vi "HFRR ADV v036 new software.vi"() -> ()   [LabVIEW 2025] (continued)
        n2892 = case shown="True" "OK Button 16" {
          frame False {
          }
          frame True {
            n2893 = stacked-sequence {
              frame #0 {
                n2894 = local read "Numeric 16"() -> (w3957:i32)
                n2895 = local write "Numeric 10"(w3957) -> ()
              }
              frame #1 {
                n2896 = local read "String 29"() -> (w3960:string)
                n2897 = String To Path(string=w3960) -> (path=w3959:path)
                n2898 = Open/Create/Replace File "Open File"(file path (use dialog)=w3959) -> (refnum out=w3961:refnum<file>)  [unwired: 5 in, 2 out]
                n2899 = for {
                  N: 16 -> [_]
                  tunnel: w3961 -> [w3968]
                  i -> [w3964]
                  (unwired) TRUE ("line mode (F)")
                  n2900 = Read from Text File "Read File"(file (use dialog)=w3968) -> (text=w3962:string)  [unwired: 3 in, 3 out]
                  n2901 = Match Pattern(string=w3962, regular expression="(") -> (after substring=w3967:string)  [unwired: 1 in, 3 out]
                  n2902 = Match Pattern(string=w3967, regular expression=")") -> (before substring=w3963:string)  [unwired: 1 in, 3 out]
                  n2903 = case shown="1" w3964 {
                    tunnel: w3963 -> [w3969 w3970 _ _ w3971 w3972 w3973 w3975 w3977 w3979 w3981 w3983 w3985 w3987 _]
                    tunnel: w3962 -> [_ _ _ _ _ _ _ _ _ _ _ _ _ _ _]
                    frame 0 {
                      "TITTLE" <- w3969
                    }
                    frame 1 {
                      "Sample ID" <- w3970
                    }
                    frame 2 {
                    }
                    frame 3 {
                    }
                    frame 4 {
                      "Test Date" <- w3971
                    }
                    frame 5 {
                      "Tested by" <- w3972
                    }
                    frame 6 {
                      n2904 = Fract/Exp String To Number(string=w3973) -> (number=→"Humidity before test 2":dbl)  [unwired: 3 in, 1 out]
                    }
                    frame 7 {
                      n2905 = Fract/Exp String To Number(string=w3975) -> (number=→"Temperature before test 2":dbl)  [unwired: 3 in, 1 out]
                    }
                    frame 8 {
                      n2906 = Fract/Exp String To Number(string=w3977) -> (number=→"Humidity after test 2":dbl)  [unwired: 3 in, 1 out]
                    }
                    frame 9 {
                      n2907 = Fract/Exp String To Number(string=w3979) -> (number=→"Temperature after test 2":dbl)  [unwired: 3 in, 1 out]
                    }
                    frame 10 {
                      n2908 = Fract/Exp String To Number(string=w3981) -> (number=→"MWSD 2":dbl)  [unwired: 3 in, 1 out]
                    }
                    frame 11 {
                      n2909 = Fract/Exp String To Number(string=w3983) -> (number=→"AVP 2":dbl)  [unwired: 3 in, 1 out]
                    }
                    frame 12 {
                      n2910 = Fract/Exp String To Number(string=w3985) -> (number=→"HCF 2":dbl)  [unwired: 3 in, 1 out]
                    }
                    frame 13 {
                      n2911 = Fract/Exp String To Number(string=w3987) -> (number=→"WS1.4 2":dbl)  [unwired: 3 in, 1 out]
                    }
                    frame 14, Default {
                    }
                  }
                }
              }
              frame #2 {
              }
            }
            n2912 = local write "OK Button 16"(FALSE ("OK Button 13")) -> ()
          }
        }
        n2913 = Index Array(array=w3632, index="Select Printer 3") -> (element=w3634:string)
        "Selected Printer" <- w3634
        n2914 = case shown="True" w3629 {
          frame False {
          }
          frame True {
            n2915 = flat-sequence {
              frame #0 {
              }
              frame #1 {
                n2916 = Wait (ms)(milliseconds to wait=u32 100) -> ()  [unwired: 1 out]
              }
              frame #2 {
                n2917 = local write "OK Button 16"(FALSE ("Print 3")) -> ()
              }
            }
          }
        }
        n2918 = case shown="True" "Print" {
          tunnel: w3634 -> [_ w3926]
          frame False {
          }
          frame True {
            (unwired) i16 6 ("width (-)")
            (unwired) "TESTED BY : "
            (unwired) "TESTED DATE :"
            (unwired) "SAMPLE ID : "
            (unwired) "SAMPLE DESIGN : "
            w3884 = "\r"
            w3901 = "\r"
            # "add image"
            n2919 = local read "Sample ID"() -> (w3874:string)
            n2920 = local read "Tested by"() -> (w3877:string)
            n2921 = local read "String 34"() -> (w3864:string)
            n2922 = local read "String 45"() -> (w3844:string)
            n2923 = local read "String 35"() -> (w3859:string)
            n2924 = local read "String 37"() -> (w3857:string)
            n2925 = local read "String 32"() -> (w3879:string)
            n2926 = local read "String 36"() -> (w3854:string)
            n2927 = local read "String 31"() -> (w3878:string)
            n2928 = local read "Test Date"() -> (w3875:string)
            n2929 = local read "String 33"() -> (w3880:string)
            n2930 = local read "String 38"() -> (w3850:string)
            n2931 = local read "String 39"() -> (w3847:string)
            n2932 = local write "Print"(FALSE ("Print FF")) -> ()
            n2933 = local read "S 39"() -> (w3862:string)
            n2934 = local read "S 38"() -> (w3869:string)
            n2935 = local read "Temperature before test 2"() -> (w3900:dbl)
            n2936 = local read "Temperature after test 2"() -> (w3890:dbl)
            n2937 = local read "Humidity before test 2"() -> (w3915:dbl)
            n2938 = local read "Humidity after test 2"() -> (w3899:dbl)
            n2939 = local read "MWSD 2"() -> (w3904:dbl)
            n2940 = local read "WS1.4 2"() -> (w3882:dbl)
            n2941 = Concatenate Strings("2)" ("string"), w3864) -> (w3865:string)
            n2942 = Concatenate Strings("3)" ("string"), w3862) -> (w3863:string)
            n2943 = Concatenate Strings("1)" ("string"), w3869) -> (w3868:string)
            n2944 = Concatenate Strings("4)" ("string"), w3859) -> (w3860:string)
            n2945 = Concatenate Strings("5)" ("string"), w3857) -> (w3856:string)
            n2946 = Concatenate Strings("6)" ("string"), w3854) -> (w3853:string)
            n2947 = Concatenate Strings("7)" ("string"), w3850) -> (w3851:string)
            n2948 = Concatenate Strings("8)" ("string"), w3847) -> (w3848:string)
            n2949 = local read "HCF 2"() -> (w3886:dbl)
            n2950 = local read "AVP 2"() -> (w3903:dbl)
            n2951 = local read "s.NO"() -> (w3845:string)
            n2952 = call <vilib>:"New Report.vi"("report type"=enum16{"Standard Report", "HTML"}."Standard Report") -> ("report out"=w3924:refnum<class "NI_report.lvclass">, "error out"=w3923:errorcluster)  [unwired: 13 in]
            n2953 = local read "TITTLE"() -> (w3876:string)
            n2954 = Concatenate Strings(w3901, w3844, w3845, w3901, w3879, w3874, w3901, w3878, w3875, w3901, w3880, w3877, w3901) -> (w3894:string)
            "test by" <- w3894
            n2955 = Number To Fractional String(number=w3900, width (-)=i16 6, precision (6)=i16 2) -> (F-format string=w3889:string)  [unwired: 1 in]
            n2956 = Number To Fractional String(number=w3899, width (-)=i16 6, precision (6)=i16 2) -> (F-format string=w3902:string)  [unwired: 1 in]
            n2957 = Number To Fractional String(number=w3915, width (-)=i16 6, precision (6)=i16 2) -> (F-format string=w3920:string)  [unwired: 1 in]
            n2958 = Number To Fractional String(number=w3904, width (-)=i16 6, precision (6)=i16 2) -> (F-format string=w3906:string)  [unwired: 1 in]
            n2959 = Number To Fractional String(number=w3890, width (-)=i16 6, precision (6)=i16 2) -> (F-format string=w3891:string)  [unwired: 1 in]
            n2960 = Number To Fractional String(number=w3903, width (-)=i16 6, precision (6)=i16 2) -> (F-format string=w3905:string)  [unwired: 1 in]
            n2961 = Number To Fractional String(number=w3886, width (-)=i16 6, precision (6)=i16 2) -> (F-format string=w3885:string)  [unwired: 1 in]
            n2962 = Number To Fractional String(number=w3882, precision (6)=i16 2) -> (F-format string=w3881:string)  [unwired: 2 in]
            n2963 = call-dynamic "Set Report Header Text.vi"("report in"=w3924, "center header text"=w3876, "error in (no error)"=w3923) -> ("report out"=w3895:refnum<class "NI_report.lvclass">, "error out"=w3896:errorcluster)  [unwired: 11 in]
            n2964 = Concatenate Strings(w3884, w3868, w3920, w3884, w3865, w3889, w3884, w3863, w3902, w3884, w3860, w3891, w3884, w3856, w3906, w3884, w3853, w3905, w3884, w3851, w3885, w3884, w3848, w3881) -> (w3872:string)
            "export 2" <- w3872
            n2965 = call-poly <vilib>:"Append Report Text.vi"("report in"=w3895, "text"=w3894, "error in (no error)"=w3896) -> ("report out"=w3898:refnum<class "NI_report.lvclass">, "error out"=w3897:errorcluster)  [unwired: 9 in, 2 out]
            n2966 = local read "test by"() -> (w3871:string)
            n2967 = local read "TITTLE"() -> (w3873:string)
            n2968 = call-poly <vilib>:"Append Report Text.vi"("report in"=w3898, "error in (no error)"=w3897) -> ("report out"=w3919:refnum<class "NI_report.lvclass">, "error out"=w3917:errorcluster)  [unwired: 10 in, 2 out]
            n2969 = Concatenate Strings(w3873, w3872, w3871) -> (→"output":string)
            n2970 = call-poly <vilib>:"Append Report Text.vi"("report in"=w3919, "text"=w3872, "error in (no error)"=w3917) -> ("report out"=w3918:refnum<class "NI_report.lvclass">, "error out"=w3916:errorcluster)  [unwired: 9 in, 2 out]
            n2971 = call-dynamic "Print Report.vi"("report in"=w3918, "printer name (default)"=w3926, "error in (no error)"=w3916) -> ("report out"=w3928:refnum<class "NI_report.lvclass">, "error out"=w3929:errorcluster)  [unwired: 11 in]
            n2972 = call-dynamic "Dispose Report.vi"("report in"=w3928, "error in (no error)"=w3929) -> ()  [unwired: 13 in, 1 out]
          }
        }
        n2973 = case shown="True" "Print 2" {
          frame False {
          }
          frame True {
            n2974 = flat-sequence {
              frame #0 {
                n2975 = local read "s.NO"() -> (→"s.NO 2":string)
                n2976 = Wait (ms)(milliseconds to wait=u32 20) -> ()  [unwired: 1 out]
                n2977 = local read "Sample ID  3"() -> (→"Sample ID  6":string)
                n2978 = local read "Sample ID  4"() -> (→"Sample ID  7":string)
                n2979 = local read "Sample ID"() -> (→"Sample ID  2":string)
                n2980 = local read "Tested by"() -> (→"Tested by 2":string)
                n2981 = local read "Test Date"() -> (→"Test Date 2":string)
                n2982 = local read "Humidity after test 3"() -> (→"Humidity after test 4":dbl)
                n2983 = local read "Ref A Test Date :"() -> (→"TITTLE 4":string)
                n2984 = local read "Temperature before test 3"() -> (w3751:dbl)
                n2985 = local read "Temperature before test 3"() -> (→"Temperature after test 5":dbl)
                n2986 = local read "Temperature after test 3"() -> (→"Temperature after test 4":dbl)
                n2987 = local read "Humidity before test 3"() -> (→"Humidity before test 4":dbl)
                n2988 = local write "Temperature before test 3"(w3751) -> ()
                n2989 = local read "image data"() -> (w3742:T16)
                n2990 = String To Path(string="C:\\LAB-IQ\\im\\Temp_resized.jpg") -> (path=w3743:path)
                "path 2" <- w3743
                n2991 = call <vilib>:"Write JPEG File.vi"("image data"=w3742, "path to JPEG file"=w3743) -> ()  [unwired: 8 in, 2 out]
                "Ref A Test Date :" <- "Ref A Test Date :"
                "Ref B Test Date :" <- "Ref B Test Date :"
                "Ref B Scar Value :" <- "Ref B Scar Value :"
                "Ref A Scar Value :" <- "Ref A Scar Value :"
              }
              frame #1 {
                (unwired) HTML_Report_Image_Alignment."MIDDLE" ("alignment (default)")
                w3779 = u16 0 items=["portrait", "landscape"] ("orientation (portrait)")
                (unwired) HTML_Report_Image_Alignment."ABSMIDDLE" ("alignment (default)")
                (unwired) "TESTED BY : "
                (unwired) "TESTED DATE :"
                (unwired) "SAMPLE ID : "
                (unwired) "SAMPLE DESIGN : "
                w3812 = "\r"
                # "add image"
                n2992 = Wait (ms)(milliseconds to wait=u32 20) -> ()  [unwired: 1 out]
                n2993 = local read "Sample ID  2"() -> (w3805:string)
                n2994 = local read "Wear Scar X"() -> (w3777:dbl)
                "Length ( microns ) 2" <- w3777
                n2995 = local read "Wear Scar Y"() -> (w3776:dbl)
                "Wear Scar Y ( microns ) :" <- w3776
                n2996 = local read "Test Date 2"() -> (w3806:string)
                n2997 = local read "Tested by 2"() -> (w3807:string)
                n2998 = local read "String 46"() -> (w3803:string)
                n2999 = local read "String 48"() -> (w3809:string)
                n3000 = local read "String 47"() -> (w3808:string)
                n3001 = local read "String 49"() -> (w3810:string)
                n3002 = local read "String 10"() -> (w3763:string)
                n3003 = local read "s.NO 2"() -> (w3804:string)
                n3004 = Add(x=w3777, y=w3776) -> (x+y=w3775:dbl)
                n3005 = call <vilib>:"New Report.vi"("report type"=enum16{"Standard Report", "HTML"}."HTML") -> ("report out"=w3783:refnum<class "NI_report.lvclass">, "error out"=w3781:errorcluster)  [unwired: 13 in]
                n3006 = Concatenate Strings(w3812, w3803, w3804, w3812, w3809, w3805, w3812, w3808, w3806, w3812, w3810, w3807, w3812) -> (→"test by 2":string)
                n3007 = Concatenate Strings("C:\\LAB-IQ\\Data\\" ("string"), w3763, ".jpg" ("string")) -> ()  [unwired: 1 out]
                n3008 = Divide(x=w3775, y=2.0) -> (x/y=→"Mean Wear ( microns) :":dbl)
                n3009 = call-dynamic "Set Report Orientation.vi"("report in"=w3783, "orientation (portrait)"=w3779, "error in (no error)"=w3781) -> ("report out"=w3782:refnum<class "NI_report.lvclass">, "error out"=w3780:errorcluster)  [unwired: 11 in]
                n3010 = for {
                  N: 5 -> [_]
                  tunnel: w3782 -> [w3833]
                  tunnel: [w3832] -> w3761
                  tunnel: w3780 -> [w3831]
                  tunnel: [w3830] -> w3760
                  n3011 = call-dynamic "Set Report Tab Width.vi"("report in"=w3833, "error in (no error)"=w3831) -> ("report out"=w3832:refnum<class "NI_report.lvclass">, "error out"=w3830:errorcluster)  [unwired: 12 in]
                }
                n3012 = local read "TITTLE"() -> (w3778:string)
                n3013 = call-dynamic "Set Report Header Text.vi"("report in"=w3761, "center header text"=w3778, "error in (no error)"=w3760) -> ("report out"=w3799:refnum<class "NI_report.lvclass">, "error out"=w3798:errorcluster)  [unwired: 11 in]
                n3014 = for {
                  N: 1 -> [_]
                  tunnel: [w3837] -> w3785
                  tunnel: [w3836] -> w3784
                  tunnel: w3799 -> [w3835]
                  tunnel: w3798 -> [w3834]
                  n3015 = call-dynamic "New Report Line.vi"("report in"=w3835, "error in (no error)"=w3834) -> ("report out"=w3837:refnum<class "NI_report.lvclass">, "error out"=w3836:errorcluster)  [unwired: 12 in]
                }
                n3016 = for {
                  N: 2 -> [_]
                  tunnel: [w3829] -> w3791
                  tunnel: [w3828] -> w3790
                  tunnel: w3785 -> [w3827]
                  tunnel: w3784 -> [w3826]
                  n3017 = call-dynamic "New Report Line.vi"("report in"=w3827, "error in (no error)"=w3826) -> ("report out"=w3829:refnum<class "NI_report.lvclass">, "error out"=w3828:errorcluster)  [unwired: 12 in]
                }
                n3018 = for {
                  N: 25 -> [_]
                  tunnel: w3791 -> [w3825]
                  tunnel: w3790 -> [w3823]
                  tunnel: [w3824] -> w3794
                  tunnel: [w3822] -> w3793
                  n3019 = call-dynamic "Set Report Tab Width.vi"("report in"=w3825, "error in (no error)"=w3823) -> ("report out"=w3824:refnum<class "NI_report.lvclass">, "error out"=w3822:errorcluster)  [unwired: 12 in]
                }
                n3020 = control-ref of="Tab Control 9"() -> (w3789:refnum<vi>)
                n3021 = call-dynamic "Append Control Image to Report.vi"("report in"=w3794, "alignment (default)"=HTML_Report_Image_Alignment."ABSMIDDLE", "ctrl reference"=w3789, "error in (no error)"=w3793) -> ("report out"=w3788:refnum<class "NI_report.lvclass">, "error out"=w3787:errorcluster)  [unwired: 8 in, 2 out]
                n3022 = for {
                  N: 3 -> [_]
                  tunnel: [w3821] -> w3772
                  tunnel: [w3820] -> w3771
                  tunnel: w3788 -> [w3819]
                  tunnel: w3787 -> [w3818]
                  n3023 = call-dynamic "New Report Line.vi"("report in"=w3819, "error in (no error)"=w3818) -> ("report out"=w3821:refnum<class "NI_report.lvclass">, "error out"=w3820:errorcluster)  [unwired: 12 in]
                }
                n3024 = for {
                  N: 100 -> [_]
                  tunnel: w3772 -> [w3817]
                  tunnel: w3771 -> [w3815]
                  tunnel: [w3816] -> w3768
                  tunnel: [w3814] -> w3766
                  n3025 = call-dynamic "Set Report Tab Width.vi"("report in"=w3817, "error in (no error)"=w3815) -> ("report out"=w3816:refnum<class "NI_report.lvclass">, "error out"=w3814:errorcluster)  [unwired: 12 in]
                }
                n3026 = String To Path(string="C:\\LAB-IQ\\im\\Temp_resized.jpg") -> (path=w3758:path)
                n3027 = call-poly <vilib>:"Append Image to Report.vi"("report in"=w3768, "path or URL of image"=w3758, "error in (no error)"=w3766) -> ("report out"=w3767:refnum<class "NI_report.lvclass">, "error out"=w3765:errorcluster)  [unwired: 9 in, 2 out]
                n3028 = call-poly <vilib>:"Open HTML Report in Browser.vi"("report in"=w3767, "error in (no error)"=w3765) -> ("report out"=w3802:refnum<class "NI_report.lvclass">, "error out"=w3801:errorcluster)  [unwired: 11 in, 1 out]
                n3029 = call-dynamic "Dispose Report.vi"("report in"=w3802, "error in (no error)"=w3801) -> ()  [unwired: 13 in, 1 out]
              }
              frame #2 {
              }
              frame #3 {
                n3030 = disable-structure shown="Disabled" {
                  frame Disabled {
                    n3031 = local read "String 10"() -> (w3842:string)
                    n3032 = Concatenate Strings("C:\\LAB-IQ-NXT\\Data\\" ("string"), w3842, ".jpg" ("string")) -> (w3840:string)
                    n3033 = String To Path(string=w3840) -> (path=w3839:path)
                    n3034 = Delete(path (use dialog)=w3839) -> ()  [unwired: 4 in, 3 out]
                  }
                  frame Enabled {
                  }
                }
                n3035 = local write "Print 2"(FALSE ("Print")) -> ()
              }
            }
          }
        }
      }
    }
    n3036 = Wait (ms)(milliseconds to wait=u32 50) -> ()  [unwired: 1 out]
    n3037 = Wait (ms)(milliseconds to wait=u32 50) -> ()  [unwired: 1 out]
    n3038 = local read "Quit"() -> (w2176:bool)
  }
  n3039 = VISA Close(VISA resource name=w41, error in (no error)=w40) -> ()  [unwired: 1 out]
  n3040 = while {
    stop <- w3993 stop-if-true
    n3041 = local read "Auto Start Test"() -> (w3991:bool)
    n3042 = local read "RUN"() -> (w3990:bool)
    n3043 = Wait (ms)(milliseconds to wait=u32 1000) -> ()  [unwired: 1 out]
    n3044 = Or(x=w3990, y=w3991) -> (x .or. y?=w3989:bool)
    n3045 = case shown="True" w3989 {
      frame False {
      }
      frame True {
        n3046 = local read "LVDT STROKE Actual"() -> (w3994:dbl)
        n3047 = In Range and Coerce(upper limit=1.2, x=w3994, lower limit=0.6) -> (In Range?=w3997:bool)  [unwired: 1 out]
        n3048 = call-poly <vilib>:"Random Number (Range).vi"("lower bound (0)"=0.998 ("upper bound (100)"), "upper bound (100)"=1.003) -> ("number"=w3995:dbl)  [unwired: 9 in]
        n3049 = case shown="True" w3997 {
          tunnel: [w4002 w4003] -> w3996
          tunnel: w3995 -> [_ w4003]
          tunnel: w3994 -> [w4002 _]
          frame False {
          }
          frame True {
          }
        }
        "LVDT STROKE DISPLAY" <- w3996
      }
    }
    n3050 = local read "Quit"() -> (w3993:bool)
  }
  n3051 = while {
    tunnel: [w4020] -> w49
    shift-right: [w4013] -> _
    shift-left: 0.0 -> [w4016]
    shift-right: [w4012] -> _
    shift-left: 0.0 -> [w4015]
    shift-right: [w4011] -> _
    shift-left: 100.0 ("vc_cmd") -> [w4014]
    stop <- w4020 stop-if-true
    # "PID LOGIC"
    n3052 = local read "run test Calibration"() -> (w4008:bool)
    n3053 = local read "RUN"() -> (w4018:bool)
    n3054 = local read "Auto Start Temp"() -> (w4009:bool)
    n3055 = local read "Auto Start Test"() -> (w4017:bool)
    n3056 = local read "START TEMP"() -> (w4007:bool)
    n3057 = And(x=w4009, y=w4017) -> (x .and. y?=w4010:bool)
    n3058 = Or(x=w4018, y=w4010) -> (x .or. y?=w4019:bool)
    n3059 = And(x=w4019, y=w4007) -> (x .and. y?=w4006:bool)
    n3060 = And(x=w4008, y=w4007) -> (x .and. y?=w4005:bool)
    n3061 = Or(x=w4005, y=w4006) -> (x .or. y?=w4004:bool)
    n3062 = Wait (ms)(milliseconds to wait="milliseconds to wait") -> ()  [unwired: 1 out]
    n3063 = case shown="True" w4004 {
      tunnel: [400.0 ("out_vc_cmd") w4039] -> w4011
      tunnel: [w4023 w4041] -> w4012
      tunnel: [w4023 w4040] -> w4013
      tunnel: w4016 -> [_ w4030]
      tunnel: w4015 -> [_ w4029]
      tunnel: w4014 -> [_ w4028]
      tunnel: w4008 -> [_ w4024]
      frame False {
        w4023 = 0.0 ("error_out")
      }
      frame True {
        n3064 = case shown="True" w4024 {
          tunnel: [w4048 1.0] -> w4026
          frame False {
            n3065 = local read "Set Strk"() -> (w4047:dbl)
            n3066 = Add(x=w4047, y="Add up Stroke") -> (x+y=w4048:dbl)
          }
          frame True {
          }
        }
        n3067 = local read "LVDT STROKE"() -> (w4025:dbl)
        n3068 = formula code="// Zero-Hardcode Explicit Positional-Form PID Engine\n// Inputs: target_stroke, measured_stroke, dt, prev_error, integral_accumulator_in, prev_vc_cmd\n//         kp, ki, kd, max_step_change, max_amplitude, min_amplitude, startup_cmd\n// Outputs: vc_cmd, error_out, out_error, integral_accumulator_out, out_vc_cmd\n\n// 1. Calculate Tracking Error\nfloat current_error = target_stroke - measured_stroke;\nerror_out = current_error;\n\n// 2. Compute Proportional Term\nfloat p_term = kp * current_error;\n\n// 3. Compute Derivative Term\nfloat d_term = 0.0;\nif (dt > 0.0) {\n    d_term = kd * ((current_error - prev_error) / dt);\n}\n\n// 4. Update and Accumulate Integral Term\nfloat current_integral = integral_accumulator_in + (current_error * dt);\nfloat i_term = ki * current_integral;\n\n// 5. Calculate Ideal Target Command (Anchored by startup baseline)\nfloat ideal_command = startup_cmd + p_term + i_term + d_term;\n\n// 6. Apply Loop Rate Limiting FIRST \n// (Forces the command to climb gradually from prev_vc_cmd instead of jumping straight to max)\nfloat raw_adjustment = ideal_command - prev_vc_cmd;\n\nif (raw_adjustment > max_step_change) {\n    raw_adjustment = max_step_change;\n} else if (raw_adjustment < -max_step_change) {\n    raw_adjustment = -max_step_change;\n}\n\nfloat next_vc_cmd = prev_vc_cmd + raw_adjustment;\n\n// 7. Anti-Windup Protection & Final Output Safety Safeguard Clamping\n// (Back-calculating based on what we are ACTUALLY outputting)\nif (next_vc_cmd > max_amplitude) {\n    float excess = next_vc_cmd - max_amplitude;\n    if (ki > 0.0) {\n        current_integral -= excess / ki;\n    }\n    next_vc_cmd = max_amplitude;\n} else if (next_vc_cmd < min_amplitude) {\n    float excess = next_vc_cmd - min_amplitude;\n    if (ki > 0.0) {\n        current_integral -= excess / ki;\n    }\n    next_vc_cmd = min_amplitude;\n}\n\n// 8. Map to Shift Registers for memory persistence\nvc_cmd = next_vc_cmd;\nout_error = current_error;                   \nintegral_accumulator_out = current_integral;  \nout_vc_cmd = next_vc_cmd;"("target_stroke"=w4026, "measured_stroke"=w4025, "dt"="dt", "integral_accumulator_in"=w4029, "prev_error"=w4030, "prev_vc_cmd"=w4028, "kp"="kp", "ki"="ki", "kd"="kd", "max_step_change"="max_step_change", "max_amplitude"="max_amplitude", "min_amplitude"="min_amplitude", "startup_cmd"="startup_cmd") -> ("vc_cmd"=w4045:dbl, "out_error"=w4040:dbl, "integral_accumulator_out"=w4041:dbl, "out_vc_cmd"=w4039:dbl)  [unwired: 1 out]
        "output Vpp" <- w4045
        n3069 = Number To Fractional String(number=w4045, precision (6)=i16 1) -> (F-format string=w4043:string)  [unwired: 2 in]
        n3070 = Concatenate Strings("DAC;" ("string"), w4043) -> (w4027:string)
        n3071 = local write "Due Write"(w4027) -> ()
        "prev_error" <- w4030
        "integral_accumulator_in" <- w4029
        "prev_vc_cmd" <- w4028
      }
    }
    n3072 = local read "Quit"() -> (w4020:bool)
  }
  n3073 = Or(x=w45, y=w44) -> (x .or. y?=w46:bool)
  n3074 = Or(x=w42, y=w46) -> (x .or. y?=w51:bool)
  n3075 = control-ref of="new picture"() -> ()  [unwired: 1 out]
  n3076 = Or(x=w54, y=w51) -> (x .or. y?=w48:bool)
  n3077 = Or(x=w48, y=w49) -> (x .or. y?=w43:bool)
  n3078 = while {
    tunnel: [w4050] -> w53
    i -> [w4057]
    stop <- w4050 stop-if-true
    n3079 = local read "Quit"() -> (w4050:bool)
    n3080 = Equal To 0?(x=w4057) -> (x = 0?=w4055:bool)
    n3081 = call "Elapsed Time3"("Time Target (s)"=45.0, "Auto Reset"=TRUE) -> ("Time has Elapsed"=w4054:bool)  [unwired: 10 in, 7 out]
    n3082 = Wait (ms)(milliseconds to wait=u32 50) -> ()  [unwired: 1 out]
    n3083 = Or(x=w4054, y=w4055) -> (x .or. y?=w4056:bool)
    n3084 = case shown="True" w4056 {
      frame False {
      }
      frame True {
        n3085 = call <vilib>:"System Exec.vi"("run minimized? (F)"=TRUE, "error in (no error)"="error in (no error)", "command line"="powercfg.exe -change -monitor-timeout-ac 0") -> ("error out"=w4068:errorcluster)  [unwired: 5 in, 3 out]
        n3086 = call <vilib>:"System Exec.vi"("run minimized? (F)"=TRUE, "error in (no error)"=w4068, "command line"="powercfg.exe -change -disk-timeout-ac 0") -> ("error out"=w4067:errorcluster)  [unwired: 5 in, 3 out]
        n3087 = call <vilib>:"System Exec.vi"("run minimized? (F)"=TRUE, "error in (no error)"=w4067, "command line"="powercfg.exe -change -standby-timeout-ac 0") -> ("error out"=w4066:errorcluster)  [unwired: 5 in, 3 out]
        n3088 = call <vilib>:"System Exec.vi"("run minimized? (F)"=TRUE, "error in (no error)"=w4066, "command line"="powercfg.exe -change -hibernate-timeout-ac 0") -> ("error out"=w4065:errorcluster)  [unwired: 5 in, 3 out]
        n3089 = call <vilib>:"Simple Error Handler.vi"("error in (no error)"=w4065) -> ("error out"=w4071:errorcluster)  [unwired: 4 in, 4 out]
        n3090 = call <vilib>:"Clear Errors.vi"("error in (no error)"=w4071) -> ("error out"=→"error out":errorcluster)  [unwired: 5 in, 1 out]
      }
    }
  }
  n3091 = Compound Arithmetic op=OR(w56, w43, w53) -> (w55:bool)
  n3092 = flat-sequence {
    tunnel: w55 -> [_]
    tunnel: [w4073] -> w25
    tunnel: w25 -> [_]
    frame #0 {
      n3093 = call "CLOSE CONNECTION.vi"() -> ("error out"=w4073:errorcluster)  [unwired: 11 in]
    }
    frame #1 {
      n3094 = Quit LabVIEW(quit? (T)=TRUE) -> ()
      n3095 = local write "Quit"(FALSE ("EXIT")) -> ()
    }
  }
  n3096 = property on="Heater Button" class="Bool (strict)"("Visible"=TRUE) -> ()  [unwired: 2 in, 2 out]
  n3097 = while {
    tunnel: [w4080] -> _
    i -> [w4080]
    stop <- w4076 stop-if-true
    # "Langauage selection"
    n3098 = Equal?(x="Lan flag", y=22.0) -> ()  [unwired: 1 out]
    n3099 = disable-structure shown="Disabled" {
      frame Disabled {
        n3100 = stacked-sequence {
          frame #0 {
            n3101 = case shown="\"Russian\"" "Language Selection" {
              tunnel: [0 1] -> w4082
              frame "English", Default {
              }
              frame "Russian" {
              }
            }
            n3102 = for {
              N: 130 -> [_]
              tunnel: "Table" -> [w4091]
              tunnel: w4082 -> [w4090]
              i -> [w4089]
              n3103 = Index Array(array=w4091, index (row)=w4089, index (col)=w4090) -> (element=w4088:string)
              n3104 = case shown="1" w4089 {
                tunnel: w4088 -> [w4092 w4093 _ w4094 w4095 w4096 w4097 w4098 w4099 w4100 w4101 w4102 w4103 w4104 w4105 w4106 w4107 w4108 w4109 w4110 w4111 w4112 w4113 w4114 w4115 w4116 w4117 w4118 w4119 _ _ w4120 w4121 w4122 w4123 w4124 w4125 w4134 w4141 w4148 w4155 w4159 w4162 w4165 w4167 w4169 w4170 w4171 w4172 w4173 w4174 w4175 w4176 w4177 w4178 w4179 w4180 w4181 w4182 w4183 w4184 w4185 w4186 w4187 w4188 w4189 w4190 w4191 w4192 w4193 w4194 w4195 w4196 w4197 w4198 w4199 w4200 w4201 w4202 w4203 w4204 w4205 w4206 w4207 w4208 w4209 w4210 w4211 w4212 w4213 w4214 w4215 w4216 w4217 w4218 w4219 w4220 w4221 w4222 w4223 w4224 w4225 w4226 w4227 w4228 _ w4229 w4230 w4231 w4232 w4233 w4234 w4235 w4236 w4237 w4238 w4239 w4240 w4241 _ w4242 w4243 w4244 w4245 w4246 w4247 _]
                frame 0 {
                  n3105 = local write "S"(w4092) -> ()
                }
                frame 1 {
                  n3106 = local write "S 2"(w4093) -> ()
                }
                frame 2 {
                }
                frame 3 {
                  n3107 = local write "S 4"(w4094) -> ()
                }
                frame 4 {
                  n3108 = property on="FILE" class="Str"("Caption.Text"=w4095) -> ()  [unwired: 2 in, 2 out]
                }
                frame 5 {
                  n3109 = property on="Fuel Discription :" class="Str"("Caption.Text"=w4096) -> ()  [unwired: 2 in, 2 out]
                }
                frame 6 {
                  n3110 = property on="Remarks :" class="Str"("Caption.Text"=w4097) -> ()  [unwired: 2 in, 2 out]
                }
                frame 7 {
                  n3111 = property on="Save & Continue" class="Bool (strict)"("Boolean Text.Text"=w4098) -> ()  [unwired: 2 in, 2 out]
                }
                frame 8 {
                }
                frame 9 {
                  n3112 = property on="Set Hz" class="DigNum (strict)"("Caption.Text"=w4100) -> ()  [unwired: 2 in, 2 out]
                }
                frame 10 {
                }
                frame 11 {
                  n3113 = property on="NORMAL LOAD" class="DigNum (strict)"("Caption.Text"=w4102) -> ()  [unwired: 2 in, 2 out]
                }
                frame 12 {
                }
                frame 13 {
                  n3114 = property on="Set Temp" class="DigNum (strict)"("Caption.Text"=w4104) -> ()  [unwired: 2 in, 2 out]
                }
                frame 14 {
                  n3115 = local write "S 15"(w4105) -> ()
                }
                frame 15 {
                  n3116 = property on="Set Rh" class="DigNum (strict)"("Caption.Text"=w4106) -> ()  [unwired: 2 in, 2 out]
                }
                frame 16 {
                }
                frame 17 {
                  n3117 = local write "S 18"(w4108) -> ()
                }
                frame 18 {
                  "String 17" <- w4109
                }
                frame 19 {
                  n3118 = property on="test time" class="DigNum (strict)"("Caption.Text"=w4110) -> ()  [unwired: 2 in, 2 out]
                }
                frame 20 {
                  "String 18" <- w4111
                  "String 22" <- w4111
                }
                frame 21 {
                  n3119 = property on="Elapsed time" class="DigNum (strict)"("Caption.Text"=w4112) -> ()  [unwired: 2 in, 2 out]
                }
                frame 22 {
                  n3120 = property on="Samplingtime 2" class="DigNum (strict)"("Caption.Text"=w4113) -> ()  [unwired: 2 in, 2 out]
                }
                frame 23 {
                  "String 21" <- w4114
                }
                frame 24 {
                  n3121 = property on="Countdown" class="DigNum (strict)"("Caption.Text"=w4115) -> ()  [unwired: 2 in, 2 out]
                }
                frame 25 {
                  n3122 = property on="Countdown 2" class="DigNum (strict)"("Caption.Text"=w4116) -> ()  [unwired: 2 in, 2 out]
                }
                frame 26 {
                  n3123 = property on="Engage" class="Bool (strict)"("Boolean Text.Text"=w4117) -> ()  [unwired: 2 in, 2 out]
                }
                frame 27 {
                  n3124 = property on="Boolean  4" class="Bool (strict)"("Boolean Text.Text"=w4118) -> ()  [unwired: 2 in, 2 out]
                }
                frame 28 {
                  n3125 = property on="Test \nStatus" class="Bool (strict)"("Boolean Text.Text"=w4119) -> ()  [unwired: 2 in, 2 out]
                }
                frame 29 {
                }
                frame 30 {
                }
                frame 31 {
                }
                frame 32 {
                  n3126 = property on="RSTCOF" class="Bool"("Boolean Text.Text"=w4121) -> ()  [unwired: 2 in, 2 out]
                  n3127 = property on="RST FF" class="Bool"("Boolean Text.Text"=w4121) -> ()  [unwired: 2 in, 2 out]
                  n3128 = property on="RST TEMP" class="Bool"("Boolean Text.Text"=w4121) -> ()  [unwired: 2 in, 2 out]
                  n3129 = property on="RSTV1 3" class="Bool"("Boolean Text.Text"=w4121) -> ()  [unwired: 2 in, 2 out]
                  n3130 = property on="rstv2" class="Bool"("Boolean Text.Text"=w4121) -> ()  [unwired: 2 in, 2 out]
                  n3131 = property on="RSTV1 2" class="Bool"("Boolean Text.Text"=w4121) -> ()  [unwired: 2 in, 2 out]
                  n3132 = property on="RST CP" class="Bool"("Boolean Text.Text"=w4121) -> ()  [unwired: 2 in, 2 out]
                }
                frame 33 {
                  "S 61" <- w4122
                }
                frame 34 {
                  "String 23" <- w4123
                }
                frame 35 {
                  n3133 = property on="Rh Before" class="DigNum (strict)"("Caption.Text"=w4124) -> ()  [unwired: 2 in, 2 out]
                }
                frame 36 {
                  n3134 = Match Pattern(string=w4125, regular expression=",") -> (before substring=→"bs":string, after substring=→"as":string)  [unwired: 1 in, 2 out]
                  n3135 = property on="Rh After" class="DigNum (strict)"("Caption.Text"=w4125) -> ()  [unwired: 2 in, 2 out]
                }
                frame 37 {
                  n3136 = Match Pattern(string=w4134, regular expression=",") -> (before substring=w4133:string, after substring=w4132:string)  [unwired: 1 in, 2 out]
                  "bs" <- w4133
                  "as" <- w4132
                  n3137 = Concatenate Strings(w4133, w4132) -> (w4129:string)
                  n3138 = property on="Humidity before test 2" class="DigNum (strict)"("Caption.Text"=w4129) -> ()  [unwired: 2 in, 2 out]
                  n3139 = Concatenate Strings(w4129, "=" ("string")) -> (w4130:string)
                  n3140 = local write "S 38"(w4130) -> ()
                }
                frame 38 {
                  n3141 = Match Pattern(string=w4141, regular expression=",") -> (before substring=w4140:string, after substring=w4139:string)  [unwired: 1 in, 2 out]
                  "bs" <- w4140
                  "as" <- w4139
                  n3142 = Concatenate Strings(w4140, w4139) -> (w4136:string)
                  n3143 = property on="Humidity after test 2" class="DigNum (strict)"("Caption.Text"=w4136) -> ()  [unwired: 2 in, 2 out]
                  n3144 = Concatenate Strings(w4136, "=" ("string")) -> (w4138:string)
                  n3145 = local write "S 39"(w4138) -> ()
                }
                frame 39 {
                  n3146 = Match Pattern(string=w4148, regular expression=",") -> (before substring=w4147:string, after substring=w4146:string)  [unwired: 1 in, 2 out]
                  "bs" <- w4147
                  "as" <- w4146
                  n3147 = Concatenate Strings(w4147, w4146) -> (w4143:string)
                  n3148 = property on="Temperature before test 2" class="DigNum (strict)"("Caption.Text"=w4143) -> ()  [unwired: 2 in, 2 out]
                  n3149 = Concatenate Strings(w4143, "=" ("string")) -> (→"String 34":string)
                }
                frame 40 {
                  n3150 = Match Pattern(string=w4155, regular expression=",") -> (before substring=w4154:string, after substring=w4153:string)  [unwired: 1 in, 2 out]
                  "bs" <- w4154
                  "as" <- w4153
                  n3151 = Concatenate Strings(w4154, w4153) -> (w4150:string)
                  n3152 = property on="Temperature after test 2" class="DigNum (strict)"("Caption.Text"=w4150) -> ()  [unwired: 2 in, 2 out]
                  n3153 = Concatenate Strings(w4150, "=" ("string")) -> (→"String 35":string)
                  n3154 = property on="Temperature after test" class="DigNum (strict)"("Caption.Text"=w4150) -> ()  [unwired: 2 in, 2 out]
                }
                frame 41 {
                  n3155 = property on="AVP 2" class="DigNum (strict)"("Caption.Text"=w4159) -> ()  [unwired: 2 in, 2 out]
                  n3156 = Concatenate Strings(w4159, "=" ("string")) -> (→"String 36":string)
                }
                frame 42 {
                  n3157 = property on="MWSD 2" class="DigNum (strict)"("Caption.Text"=w4162) -> ()  [unwired: 2 in, 2 out]
                  n3158 = Concatenate Strings(w4162, "=" ("string")) -> (→"String 37":string)
                }
                frame 43 {
                  n3159 = property on="HCF 2" class="DigNum (strict)"("Caption.Text"=w4165) -> ()  [unwired: 2 in, 2 out]
                  n3160 = Concatenate Strings(w4165, "=" ("string")) -> (→"String 38":string)
                }
                frame 44 {
                  n3161 = Concatenate Strings(w4167, "=" ("string")) -> (→"String 39":string)
                  n3162 = property on="WS1.4 2" class="DigNum (strict)"("Caption.Text"=w4167) -> ()  [unwired: 2 in, 2 out]
                }
                frame 45 {
                }
                frame 46 {
                  n3163 = local write "S 47"(w4170) -> ()
                }
                frame 47 {
                  n3164 = local write "S 48"(w4171) -> ()
                }
                frame 48 {
                  n3165 = local write "S 49"(w4172) -> ()
                }
                frame 49 {
                  n3166 = local write "S 50"(w4173) -> ()
                }
                frame 50 {
                  n3167 = local write "S 51"(w4174) -> ()
                }
                frame 51 {
                  n3168 = local write "S 52"(w4175) -> ()
                }
                frame 52 {
                  n3169 = local write "S 53"(w4176) -> ()
                }
                frame 53 {
                  n3170 = local write "S 54"(w4177) -> ()
                }
                frame 54 {
                  n3171 = local write "S 55"(w4178) -> ()
                }
                frame 55 {
                  n3172 = local write "S 56"(w4179) -> ()
                }
                frame 56 {
                  n3173 = local write "S 57"(w4180) -> ()
                }
                frame 57 {
                  n3174 = local write "S 58"(w4181) -> ()
                }
                frame 58 {
                  n3175 = local write "S 59"(w4182) -> ()
                }
                frame 59 {
                  n3176 = local write "S 60"(w4183) -> ()
                }
                frame 60 {
                  n3177 = local write "S 62"(w4184) -> ()
                }
                frame 61 {
                  n3178 = local write "S 63"(w4185) -> ()
                }
                frame 62 {
                  n3179 = local write "S 64"(w4186) -> ()
                }
                frame 63 {
                  n3180 = local write "S 65"(w4187) -> ()
                }
                frame 64 {
                  n3181 = local write "S 66"(w4188) -> ()
                }
                frame 65 {
                  n3182 = local write "S 67"(w4189) -> ()
                }
                frame 66 {
                  n3183 = local write "S 68"(w4190) -> ()
                }
                frame 67 {
                  n3184 = local write "S 69"(w4191) -> ()
                }
                frame 68 {
                  n3185 = local write "S 70"(w4192) -> ()
                }
                frame 69 {
                  n3186 = local write "S 71"(w4193) -> ()
                }
                frame 70 {
                  n3187 = local write "S 72"(w4194) -> ()
                }
                frame 71 {
                  n3188 = local write "S 73"(w4195) -> ()
                }
                frame 72 {
                  n3189 = local write "S 74"(w4196) -> ()
                }
                frame 73 {
                  n3190 = local write "S 75"(w4197) -> ()
                }
                frame 74 {
                  n3191 = local write "S 76"(w4198) -> ()
                }
                frame 75 {
                  n3192 = local write "S 77"(w4199) -> ()
                }
                frame 76 {
                  n3193 = local write "S 78"(w4200) -> ()
                }
                frame 77 {
                  n3194 = local write "S 79"(w4201) -> ()
                }
                frame 79 {
                  n3195 = property on="Sample Temperature ( °C )" class="XYGraph (strict)"("Y Scale.Name Label.Text"=w4202) -> ()  [unwired: 2 in, 2 out]
                }
                frame 80 {
                  n3196 = local write "S 81"(w4203) -> ()
                  n3197 = property on="Humidity ( %RH )" class="XYGraph (strict)"("Y Scale.Name Label.Text"=w4203) -> ()  [unwired: 2 in, 2 out]
                }
                frame 78 {
                  n3198 = property on="Air Temperature  ( °C )" class="XYGraph (strict)"("X Scale.Name Label.Text"=w4204) -> ()  [unwired: 2 in, 2 out]
                  n3199 = property on="Humidity ( %RH )" class="XYGraph (strict)"("X Scale.Name Label.Text"=w4204) -> ()  [unwired: 2 in, 2 out]
                  n3200 = property on="Sample Temperature ( °C )" class="XYGraph (strict)"("X Scale.Name Label.Text"=w4204) -> ()  [unwired: 2 in, 2 out]
                  n3201 = property on="Coefficient Of Friction" class="XYGraph (strict)"("X Scale.Name Label.Text"=w4204) -> ()  [unwired: 2 in, 2 out]
                }
                frame 81 {
                  n3202 = property on="Air Temperature  ( °C )" class="XYGraph (strict)"("Y Scale.Name Label.Text"=w4205) -> ()  [unwired: 2 in, 2 out]
                }
                frame 82 {
                  n3203 = local write "S 84"(w4206) -> ()
                }
                frame 83 {
                  n3204 = local write "S 85"(w4207) -> ()
                }
                frame 84 {
                  n3205 = local write "S 86"(w4208) -> ()
                }
                frame 85 {
                  n3206 = local write "S 87"(w4209) -> ()
                }
                frame 86 {
                  n3207 = local write "S 88"(w4210) -> ()
                }
                frame 87 {
                }
                frame 88 {
                  n3208 = local write "S 90"(w4212) -> ()
                }
                frame 89 {
                  n3209 = local write "S 91"(w4213) -> ()
                }
                frame 90 {
                  n3210 = local write "S 92"(w4214) -> ()
                }
                frame 91 {
                  n3211 = local write "S 93"(w4215) -> ()
                }
                frame 92 {
                  n3212 = local write "S 94"(w4216) -> ()
                }
                frame 93 {
                  n3213 = local write "S 95"(w4217) -> ()
                }
                frame 94 {
                  n3214 = local write "S 96"(w4218) -> ()
                }
                frame 95 {
                  n3215 = local write "S 97"(w4219) -> ()
                }
                frame 96 {
                  n3216 = local write "S 98"(w4220) -> ()
                }
                frame 97 {
                  n3217 = local write "S 99"(w4221) -> ()
                }
                frame 98 {
                  n3218 = local write "S 100"(w4222) -> ()
                }
                frame 99 {
                  n3219 = local write "S 101"(w4223) -> ()
                }
                frame 100 {
                  n3220 = local write "S 102"(w4224) -> ()
                }
                frame 101 {
                  n3221 = local write "S 103"(w4225) -> ()
                }
                frame 102 {
                  n3222 = local write "S 104"(w4226) -> ()
                }
                frame 103 {
                  n3223 = local write "S 105"(w4227) -> ()
                }
                frame 104 {
                  n3224 = local write "S 106"(w4228) -> ()
                }
                frame 105 {
                }
                frame 106 {
                  n3225 = property on="OK Button 17" class="Bool (strict)"("Boolean Text.Text"=w4229) -> ()  [unwired: 2 in, 2 out]
                }
                frame 107 {
                  n3226 = property on="OK Button 16" class="Bool (strict)"("Boolean Text.Text"=w4230) -> ()  [unwired: 2 in, 2 out]
                }
                frame 108 {
                  n3227 = property on="TITTLE" class="Str"("Caption.Text"=w4231) -> ()  [unwired: 2 in, 2 out]
                }
                frame 109 {
                  "String 30" <- w4232
                }
                frame 110 {
                  n3228 = property on="Test Date" class="Str"("Caption.Text"=w4233) -> ()  [unwired: 2 in, 2 out]
                  "String 31" <- w4233
                }
                frame 111 {
                  n3229 = property on="Sample ID" class="Str"("Caption.Text"=w4234) -> ()  [unwired: 2 in, 2 out]
                  "String 32" <- w4234
                }
                frame 112 {
                  n3230 = property on="Tested by" class="Str"("Caption.Text"=w4235) -> ()  [unwired: 2 in, 2 out]
                  "String 33" <- w4235
                }
                frame 113 {
                  n3231 = property on="System Configured Printers 2" class="Arr (strict)"("Caption.Text"=w4236) -> ()  [unwired: 2 in, 2 out]
                }
                frame 114 {
                  n3232 = property on="Selected Printer" class="Str"("Caption.Text"=w4237) -> ()  [unwired: 2 in, 2 out]
                }
                frame 115 {
                  n3233 = property on="Select Printer 3" class="DigNum (strict)"("Caption.Text"=w4238) -> ()  [unwired: 2 in, 2 out]
                }
                frame 116 {
                  n3234 = property on="Print" class="Bool (strict)"("Boolean Text.Text"=w4239) -> ()  [unwired: 2 in, 2 out]
                }
                frame 117 {
                  "String 41" <- w4240
                }
                frame 118 {
                  n3235 = property on="tested by" class="Str"("Caption.Text"=w4241) -> ()  [unwired: 2 in, 2 out]
                }
                frame 119 {
                }
                frame 120 {
                  n3236 = property on="Export" class="Bool (strict)"("Boolean Text.Text"=w4242) -> ()  [unwired: 2 in, 2 out]
                }
                frame 121 {
                }
                frame 122 {
                }
                frame 123 {
                  n3237 = property on="Select File Type" class="Enum (strict)"("Caption.Text"=w4245) -> ()  [unwired: 2 in, 2 out]
                }
                frame 124 {
                  n3238 = property on="s.NO" class="Str"("Caption.Text"=w4246) -> ()  [unwired: 2 in, 2 out]
                  "String 45" <- w4246
                }
                frame 125 {
                  n3239 = property on="trip1 8" class="Bool (strict)"("Boolean Text.Text"=w4247) -> ()  [unwired: 2 in, 2 out]
                }
                frame 126, Default {
                }
              }
            }
          }
          frame #1 {
            w4255 = TRUE ("Visible")
            n3240 = local read "S 91"() -> (w4272:string)
            n3241 = local read "S 90"() -> (w4271:string)
            n3242 = local read "S 88"() -> (w4270:string)
            n3243 = property on="File Path" class="Path"("Caption.Text"=w4271) -> ()  [unwired: 2 in, 2 out]
            n3244 = local read "S 71"() -> (w4265:string)
            n3245 = local read "S 86"() -> (w4267:string)
            n3246 = local read "S 85"() -> (w4268:string)
            n3247 = local read "S 87"() -> (w4266:string)
            n3248 = local read "S 84"() -> (w4269:string)
            n3249 = local read "S 103"() -> (w4254:string)
            n3250 = local read "S 104"() -> (w4253:string)
            n3251 = property on="Password" class="Str"("Caption.Text"=w4268) -> ()  [unwired: 2 in, 2 out]
            n3252 = property on="EDIT" class="Bool (strict)"("Boolean Text.Text"=w4265) -> ()  [unwired: 2 in, 2 out]
            n3253 = property on="SAVE" class="Bool (strict)"("Boolean Text.Text"=w4269) -> ()  [unwired: 2 in, 2 out]
            n3254 = Build Array(w4254, w4253) -> (w4252:string[])
            n3255 = property on="Heater Button" class="Bool (strict)"("Strings [4]"=w4252) -> ()  [unwired: 2 in, 2 out]
            n3256 = local read "S 92"() -> (w4264:string)
            n3257 = local read "S 93"() -> (w4263:string)
            n3258 = local read "S 105"() -> (w4250:string)
            n3259 = local read "S 106"() -> (w4249:string)
            n3260 = Build Array(w4264, w4263) -> ()  [unwired: 1 out]
            n3261 = Build Array(w4250, w4249) -> (w4251:string[])
            n3262 = local read "S 95"() -> (w4261:string)
            n3263 = local read "S 94"() -> (w4262:string)
            n3264 = local read "bs"() -> (w4277:string)
            n3265 = local read "as"() -> (w4278:string)
            n3266 = property on="Humidity" class="Bool (strict)"("Strings [4]"=w4251) -> ()  [unwired: 2 in, 2 out]
            n3267 = Concatenate Strings(w4277, "\r", w4278) -> ()  [unwired: 1 out]
            n3268 = property on="Rh After" class="DigNum (strict)"("Caption.Size to Text?"=TRUE ("Caption.Size to Text")) -> ()  [unwired: 2 in, 2 out]
            n3269 = local read "S 48"() -> (w4301:string)
            n3270 = local read "S 50"() -> (w4299:string)
            n3271 = local read "S 51"() -> (w4298:string)
            n3272 = local read "S 49"() -> (w4300:string)
            n3273 = local read "S 52"() -> (w4297:string)
            n3274 = local read "as"() -> (w4282:string)
            n3275 = local read "bs"() -> (w4283:string)
            n3276 = local read "S 56"() -> (w4296:string)
            n3277 = local read "S 57"() -> (w4295:string)
            n3278 = local read "S 58"() -> (w4294:string)
            n3279 = local read "S 59"() -> (w4293:string)
            n3280 = property on="OPEN" class="Bool (strict)"("Boolean Text.Text"=w4297) -> ()  [unwired: 2 in, 2 out]
            n3281 = property on="OPEN 1" class="Bool (strict)"("Boolean Text.Text"=w4301) -> ()  [unwired: 2 in, 2 out]
            n3282 = property on="OPEN 2" class="Bool (strict)"("Boolean Text.Text"=w4300) -> ()  [unwired: 2 in, 2 out]
            n3283 = property on="OPEN 3" class="Bool (strict)"("Boolean Text.Text"=w4299) -> ()  [unwired: 2 in, 2 out]
            n3284 = property on="OPEN 4" class="Bool (strict)"("Boolean Text.Text"=w4298) -> ()  [unwired: 2 in, 2 out]
            n3285 = Concatenate Strings(w4283, "\r", w4282) -> ()  [unwired: 1 out]
            n3286 = local read "S 102"() -> (w4256:string)
            n3287 = property on="КОФ1" class="DigNum (strict)"("Caption.Text"=w4296) -> ()  [unwired: 2 in, 2 out]
            n3288 = local read "S 98"() -> (w4260:string)
            n3289 = local read "S 99"() -> (w4259:string)
            n3290 = local read "S 100"() -> (w4258:string)
            n3291 = local read "S 101"() -> (w4257:string)
            n3292 = property on="КОФ2" class="DigNum (strict)"("Caption.Text"=w4295) -> ()  [unwired: 2 in, 2 out]
            n3293 = property on="КОФ3" class="DigNum (strict)"("Caption.Text"=w4294) -> ()  [unwired: 2 in, 2 out]
            n3294 = property on="КОФ4" class="DigNum (strict)"("Caption.Text"=w4293) -> ()  [unwired: 2 in, 2 out]
            n3295 = local read "bs"() -> (w4281:string)
            n3296 = local read "as"() -> (w4280:string)
            n3297 = local read "S 60"() -> (w4292:string)
            n3298 = local read "S 54"() -> (w4302:string)
            n3299 = Concatenate Strings(w4281, "\r", w4280) -> ()  [unwired: 1 out]
            n3300 = Concatenate Strings(w4302, w4292) -> ()  [unwired: 1 out]
            n3301 = local read "S 77"() -> (→"String 43":string)
            n3302 = local read "S 76"() -> (w4275:string)
            n3303 = local read "S 78"() -> (w4274:string)
            n3304 = local read "S 71"() -> (w4286:string)
            n3305 = local read "S 66"() -> (w4291:string)
            n3306 = local read "S 67"() -> (w4290:string)
            n3307 = local read "S 68"() -> (w4289:string)
            n3308 = local read "S 69"() -> (w4288:string)
            n3309 = local read "S 70"() -> (w4287:string)
            n3310 = property on="AIR TEMP" class="DigNum (strict)"("Caption.Text"=w4274) -> ()  [unwired: 2 in, 2 out]
            n3311 = property on="Set Strk" class="DigNum (strict)"("Caption.Text"=w4275) -> ()  [unwired: 2 in, 2 out]
            n3312 = property on="SPEED OUT:" class="DigNum (strict)"("Caption.Text"=w4289) -> ()  [unwired: 2 in, 2 out]
            n3313 = property on="EDIT" class="Bool (strict)"("Boolean Text.Text"=w4286) -> ()  [unwired: 2 in, 2 out]
            n3314 = local read "S 79"() -> (w4273:string)
          }
          frame #2 {
          }
        }
        n3315 = local write "Lan flag"(10.0 ("Lan flag")) -> ()
      }
      frame Enabled {
      }
    }
    n3316 = Wait (ms)(milliseconds to wait=u32 2000) -> ()  [unwired: 1 out]
    n3317 = local read "Quit"() -> (w4076:bool)
  }
  n3318 = while {
    shift-right: [w4308] -> _
    shift-left: _ -> [w4309]
    shift-right: [w4306] -> _
    shift-left: T18 {"Read Heave and Surge"="", "Bytes at Heave Port"=0.0, "Heave and Surge COM Port:"="COM9", "Com Port 2"="COM7", "Residual Due"="", "Heave COM Status 2"=TRUE, "Heave COM Status"=TRUE, "Port 2"=TRUE, "Sway PPR"=6400.0, "Surge PPR"=6400.0, "Heave PPR"=6400.0, "Sway Pitch"=2.0, "Surge Pitch"=3.0, "Heave Pitch"=4.0, "Sway Pulses/mm"=320.0, "Surge Pulses/mm"=1600.0, "Heave Pulses/mm"=1600.0, "inner loop"=0.0, "Read Heave and Surge 2"="", "String 36"="", "Write S"=FALSE, "WriteCC1"=[""], "Heave COM Loop"=0, "LastCom"="", "EXIT"=FALSE, "Error Heave"={"status"=TRUE, "code"=-1073807343, "source"=""}} -> [w4305]
    shift-right: [w4303] -> _
    shift-left: enum16{"init", "MAIN", "Panel Close"}."init" -> [w4304]
    stop <- w4307 stop-if-true
    # "HUMIDITY LOOP LOGIC"
    n3319 = case shown="\"MAIN\"" w4304 {
      tunnel: w4309 -> [w4323 w4342 w4397 w4399]
      tunnel: [w4318 w4346 w4397 w4399] -> w4308
      tunnel: [_ _ TRUE _] -> w4307
      tunnel: [w4315 w4344 w4395 w4398] -> w4306
      tunnel: w4305 -> [w4320 w4341 w4395 w4398]
      tunnel: [enum16{"init", "MAIN", "Panel Close"}."MAIN" w4336 _ _] -> w4303
      frame "init" {
        n3320 = local read "C3 :"() -> (w4310:refnum<visa-resource-name>)
        n3321 = Bundle By Name(cluster=w4320, "Heave and Surge COM Port:"=w4310) -> (w4319:T18)
        n3322 = call "Instrument fgv uno.vi"("Enum"=T31."INIT", "error in (no error) 2"=w4323, "INPUT"=w4319) -> ("error"=w4321:errorcluster, "output"=w4317:T18)  [unwired: 6 in, 1 out]
        n3323 = case shown="Error" w4321 {
          selector: w4321 -> [w4325 _]
          tunnel: [w4325 w4329] -> w4318
          tunnel: w4317 -> [w4324 w4327]
          tunnel: [w4324 w4326] -> w4316
          frame No Error {
          }
          frame Error {
            n3324 = call "Instrument fgv uno.vi"("Enum"=T31."ERROR INIT", "INPUT"=w4327) -> ("error"=w4330:errorcluster, "output"=w4326:T18)  [unwired: 7 in, 1 out]
            n3325 = call <vilib>:"Clear Errors.vi"("error in (no error)"=w4330) -> ("error out"=w4329:errorcluster)  [unwired: 5 in, 1 out]
          }
        }
        n3326 = local read "LastCom Humidity"() -> (w4313:string)
        n3327 = Unbundle By Name(w4316) -> ("Heave COM Status 2"=→"COM Status":bool, "Error Heave"=→"Error":errorcluster)  [unwired: 1 out]
        n3328 = Bundle By Name(cluster=w4316, "LastCom"=w4313) -> (w4315:T18)
      }
      frame "MAIN" {
        n3329 = Unbundle By Name(w4341) -> ("Com Port 2"=w4331:refnum<visa-resource-name>)
        n3330 = local read "C3 :"() -> (w4332:refnum<visa-resource-name>)
        n3331 = local write "COM Port Humidity :"(w4331) -> ()
        n3332 = Bundle By Name(cluster=w4341, "Heave and Surge COM Port:"=w4332) -> (w4340:T18)
        n3333 = Equal?(x=w4331, y=w4332) -> (x = y?=w4347:bool)
        n3334 = case shown="True" w4347 {
          tunnel: [w4351 w4368] -> w4346
          tunnel: w4342 -> [w4352 w4374]
          tunnel: w4340 -> [w4350 w4372]
          tunnel: [w4349 w4367] -> w4344
          frame False {
            n3335 = call <vilib>:"Clear Errors.vi"("error in (no error)"=w4352) -> ("error out"=w4348:errorcluster)  [unwired: 5 in, 1 out]
            n3336 = call "Instrument fgv uno.vi"("Enum"=T31."ERROR INIT", "error in (no error) 2"=w4348, "INPUT"=w4350) -> ("error"=w4354:errorcluster, "output"=w4349:T18)  [unwired: 6 in, 1 out]
            n3337 = call <vilib>:"Clear Errors.vi"("error in (no error)"=w4354) -> ("error out"=w4351:errorcluster)  [unwired: 5 in, 1 out]
          }
          frame True {
            n3338 = call "Instrument fgv uno.vi"("Enum"=T31."READ", "error in (no error) 2"=w4374, "INPUT"=w4372) -> ("error"=w4373:errorcluster, "output"=w4366:T18)  [unwired: 6 in, 1 out]
            n3339 = Bundle By Name(cluster=w4366, "String 36"="WRITE HUMIDITY") -> (w4365:T18)
            n3340 = case shown="True" "Write Humidity" {
              selector: "Write Humidity" -> [_ w4394]
              tunnel: w4373 -> [w4387 w4393]
              tunnel: [w4387 w4392] -> w4363
              tunnel: w4365 -> [w4386 w4390]
              tunnel: [w4386 w4389] -> w4362
              frame False {
              }
              frame True {
                n3341 = Not(x=w4394) -> (.not. x?=w4388:bool)
                n3342 = local write "Write Humidity"(w4388) -> ()
                n3343 = call "Instrument fgv uno.vi"("Enum"=T31."MANUAL WRITE", "error in (no error) 2"=w4393, "INPUT"=w4390) -> ("error"=w4392:errorcluster, "output"=w4389:T18)  [unwired: 6 in, 1 out]
              }
            }
            n3344 = Array Size(array="WriteHumidity") -> (size(s)=w4360:i32)
            n3345 = Greater Than 0?(x=w4360) -> (x > 0?=w4359:bool)
            n3346 = call "Instrument fgv uno.vi"("Enum"=T31."WRITE", "error in (no error) 2"=w4363, "WriteCC1"="WriteHumidity", "INPUT"=w4362) -> ("error"=w4370:errorcluster, "WriteCC1 2"=w4361:string[], "output"=w4369:T18)  [unwired: 5 in]
            n3347 = case shown="True" w4359 {
              tunnel: w4361 -> [_ w4376]
              frame False {
              }
              frame True {
                n3348 = local write "WriteHumidity"(w4376) -> ()
              }
            }
            n3349 = case shown="No Error" w4370 {
              selector: w4370 -> [w4377 w4380]
              tunnel: w4369 -> [w4378 w4385]
              tunnel: [w4378 w4384] -> w4367
              tunnel: [w4377 w4382] -> w4368
              frame No Error {
              }
              frame Error {
                n3350 = call <vilib>:"Clear Errors.vi"("error in (no error)"=w4380) -> ("error out"=w4379:errorcluster)  [unwired: 5 in, 1 out]
                n3351 = call "Instrument fgv uno.vi"("Enum"=T31."ERROR INIT", "error in (no error) 2"=w4379, "INPUT"=w4385) -> ("error"=w4383:errorcluster, "output"=w4384:T18)  [unwired: 6 in, 1 out]
                n3352 = call <vilib>:"Clear Errors.vi"("error in (no error)"=w4383) -> ("error out"=w4382:errorcluster)  [unwired: 5 in, 1 out]
              }
            }
            n3353 = Unbundle By Name(w4367) -> ("LastCom"=→"LastCom Humidity":string, "Read Heave and Surge"=→"Read HUMIDITY":string)
          }
        }
        n3354 = Unbundle By Name(w4344) -> ("Heave COM Status 2"=w4345:bool, "Error Heave"=w4333:errorcluster, "Bytes at Heave Port"=→"Bytes at Humidity Port  2":dbl)  [unwired: 1 out]
        n3355 = Unbundle By Name(w4333) -> ("status"=→"Humidity Port":bool)
        n3356 = Not(x=w4345) -> (.not. x?=w4334:bool)
        n3357 = local write "Error"(w4333) -> ()
        n3358 = local read "Quit"() -> (w4337:bool)
        n3359 = local write "COM Status"(w4334) -> ()
        n3360 = Select(t=enum16{"init", "MAIN", "Panel Close"}."Panel Close", s=w4337, f=enum16{"init", "MAIN", "Panel Close"}."MAIN") -> (s? t:f=w4336:enum16{"init", "MAIN", "Panel Close"})
      }
      frame "Panel Close" {
      }
      frame Default {
      }
    }
  }
  n3361 = while {
    stop <- w4402 stop-if-true
    n3362 = call <vilib>:"High Resolution Polling Wait.vi"("seconds to wait"=0.05) -> ()  [unwired: 10 in, 1 out]
    n3363 = disable-structure shown="Disabled" {
      disable-tunnel: [_ w4433] -> w4400
